vi "GUI.vi"() -> ()   [LabVIEW 2021]
uses:
  UI Data.ctl
  Data.ctl
  <vilib>/Instr/_visa.llb/VISA Configure Serial Port (Instr).vi
  styles/colors.vi
panel:
  in  "Stop button":bool
  in  "Run button":bool
  in  "Settings button":bool
  out "Console":string
  in  "Serial communication\n settings":T1={"COM"="", "baud rate"=115200, "data bits"=8, "parity"=enum."None", "stop bits"=10, "flow control"=enum."None", "delay"=50} {"stop bits" items=["1.0"=10, "1.5"=15, "2.0"=20]; "baud rate" max=921600; "data bits" max=16}
  in  "Paths":bool
  in  "Save button":bool
  in  "Path: 4.9.12.XXXX":path=path "C:/Users/ken_X/Documents/LabVIEW projects/Project-A/outset-medical/4.9.12.6034"
  in  "Path: Android OS":path=path "C:/Users/ken_X/Documents/LabVIEW projects/Project-A/outset-medical/Android OS"
  # "Serial communication\n settings"
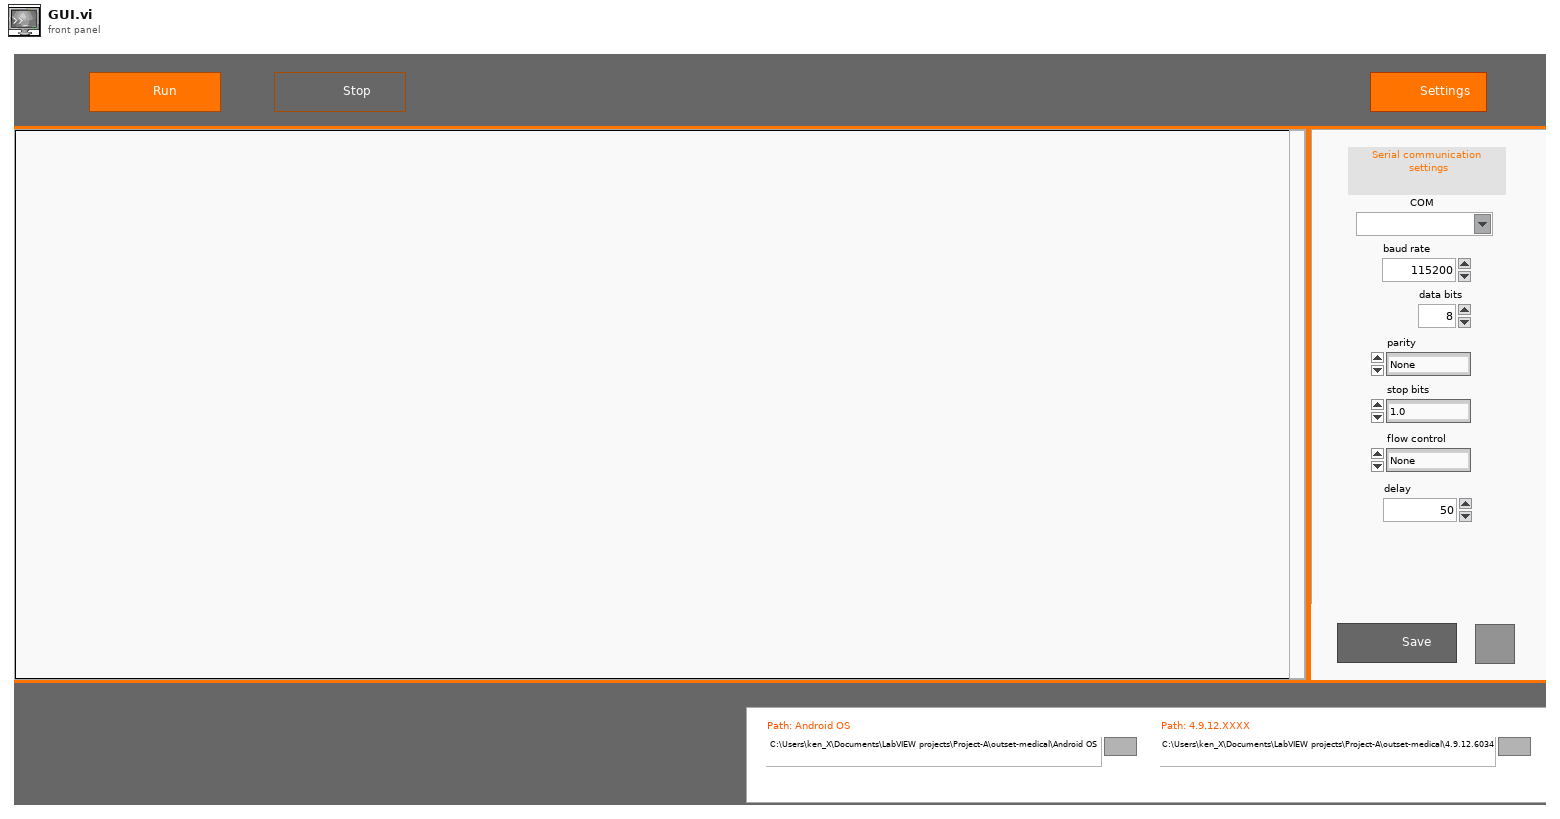
[diagram p1: front panel]
types:
  T1 = cluster{"COM":refnum<visa-resource-name>, "baud rate":u32, "data bits":u8, "parity":enum16{"None", "Odd", "Even", "Mark", "Space"}, "stop bits":u16, "flow control":enum16{"None", "XON/XOFF", "RTS/CTS", "DTR/DSR"}, "delay":u16}
  T2 = typedef "Data.ctl" = cluster{"Console":refnum<vi>, "COM":refnum<visa-resource-name>, "delay":u32, "error in":errorcluster}
  T3 = enum8{"Enabled", "Disabled", "Disabled and Grayed Out"}
  T4 = typedef "UI Data.ctl" = cluster{"settings splitter":refnum<vi>, "footer splitter":refnum<vi>, "Serial communication\n settings":refnum<vi>, "Path: Android OS":refnum<vi>, "Path: 4.9.12.XXXX":refnum<vi>}
  T5 = cluster{"primary color":u32, "secondary color":u32, "accent color":u32, "background color":u32, "accent s color":u32}
  T6 = cluster{"accent s color":u32, "accent s color":u32}
  T7 = cluster{"accent s color":u32, "accent color":u32}
  T8 = cluster{"primary color":u32, "primary color":u32}
  T9 = cluster{"secondary color":u32, "secondary color":u32}
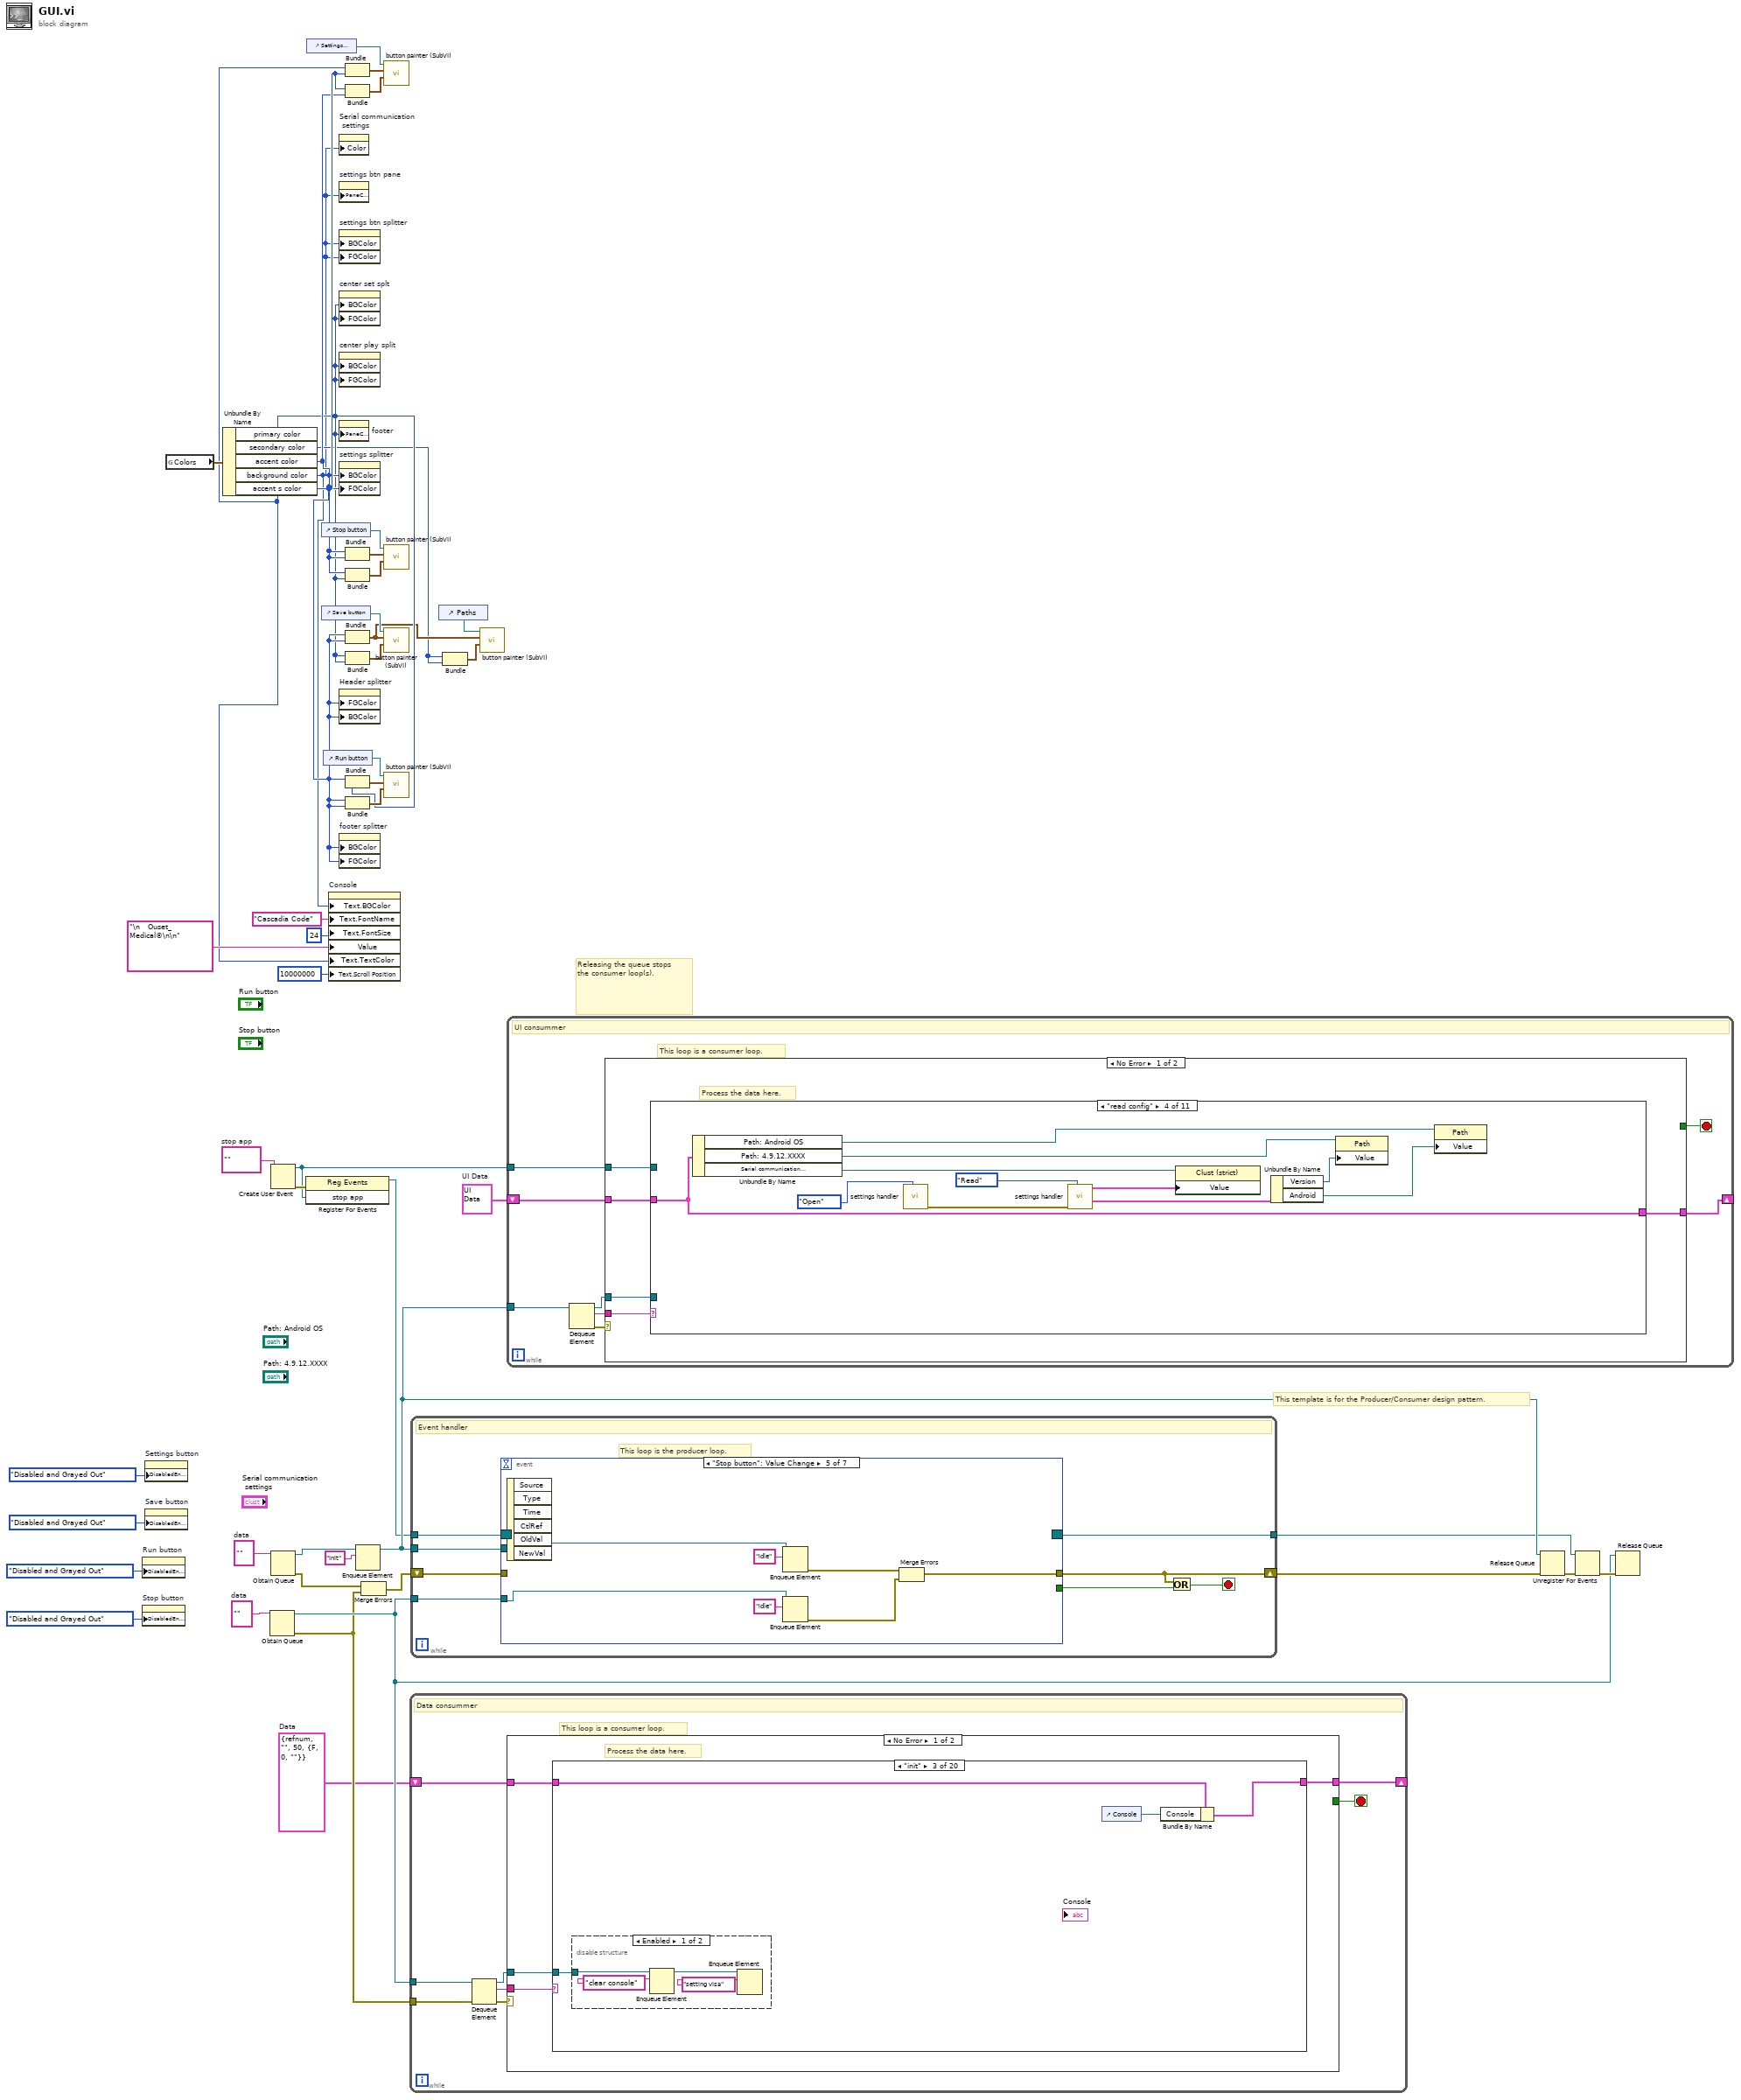
[diagram p0: block diagram]
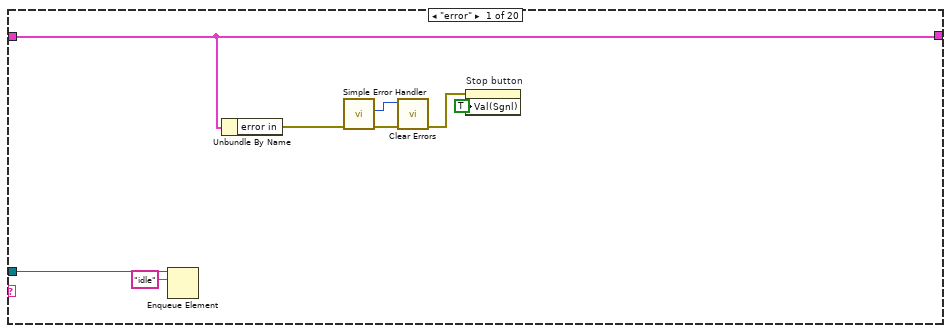
[diagram p2: hidden frame]
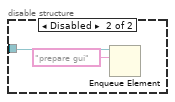
[diagram p4: hidden frame]
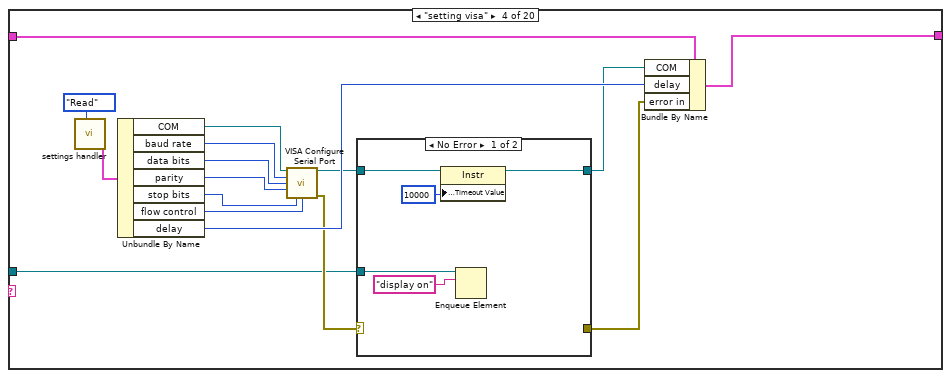
[diagram p5: hidden frame]
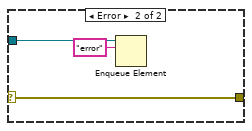
[diagram p6: hidden frame]
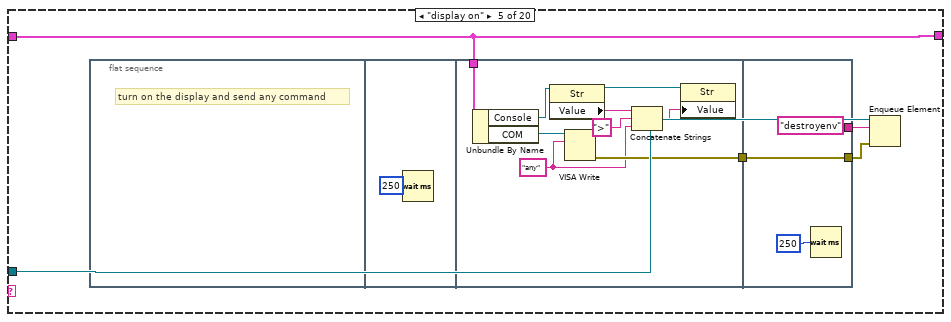
[diagram p7: hidden frame]
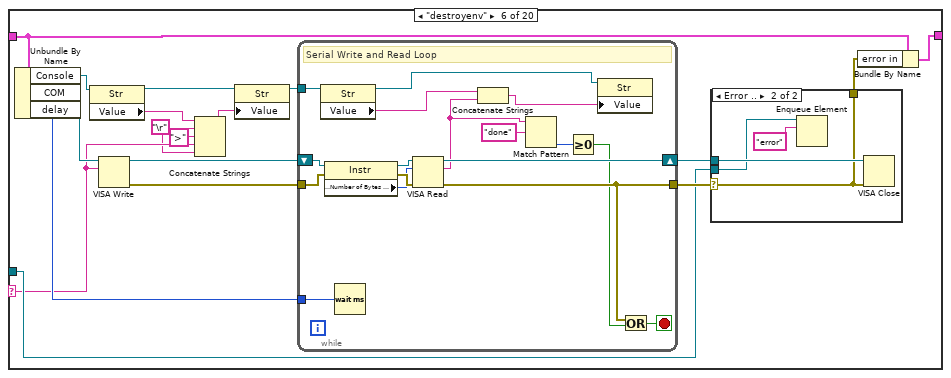
[diagram p8: hidden frame]
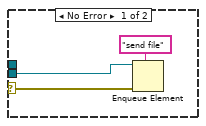
[diagram p9: hidden frame]
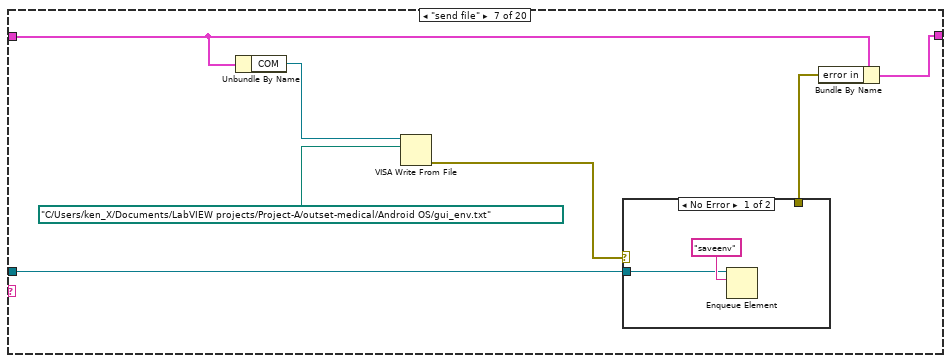
[diagram p10: hidden frame]
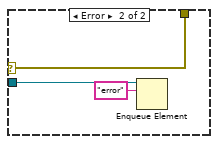
[diagram p11: hidden frame]
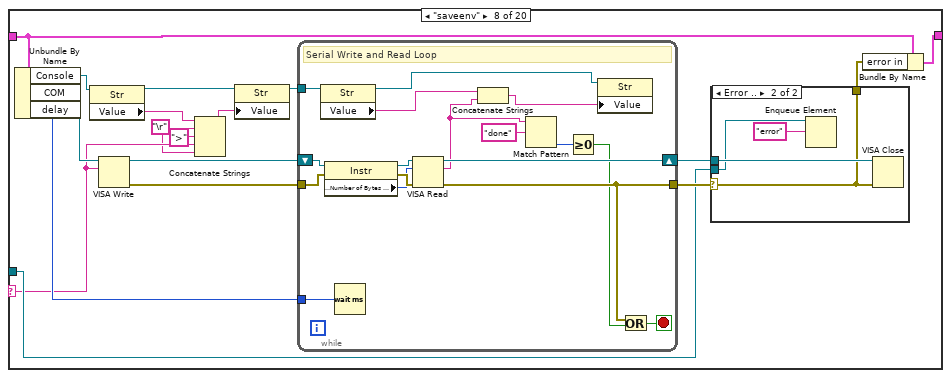
[diagram p12: hidden frame]
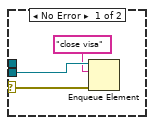
[diagram p13: hidden frame]
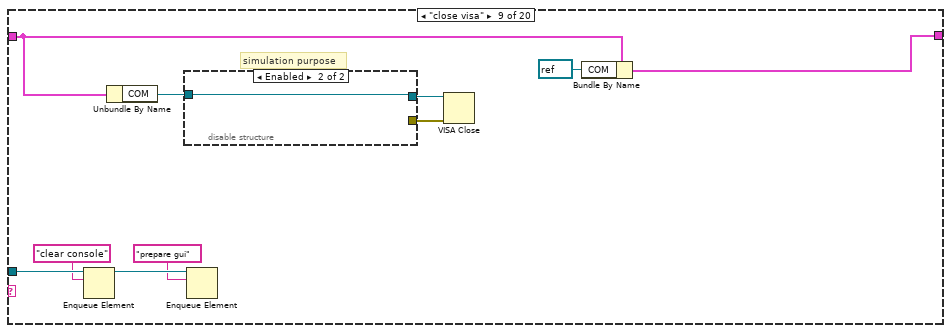
[diagram p14: hidden frame]
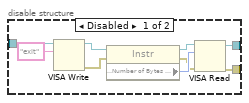
[diagram p15: hidden frame]
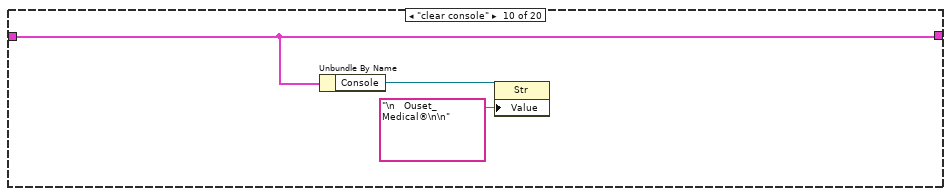
[diagram p16: hidden frame]
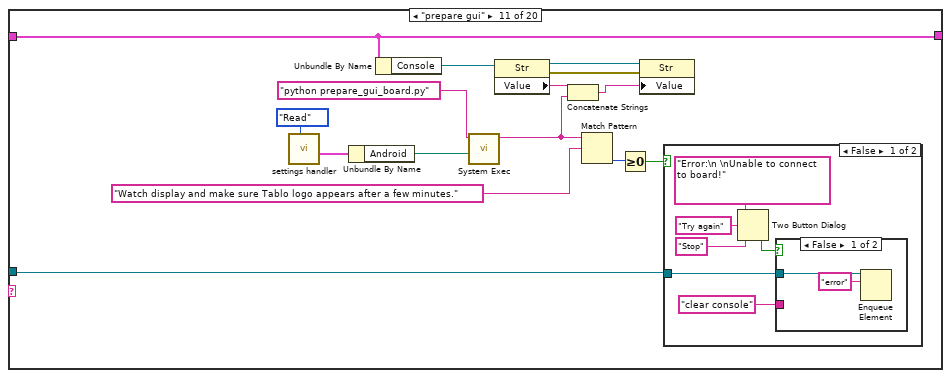
[diagram p17: hidden frame]
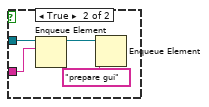
[diagram p18: hidden frame]
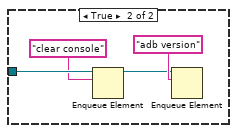
[diagram p19: hidden frame]
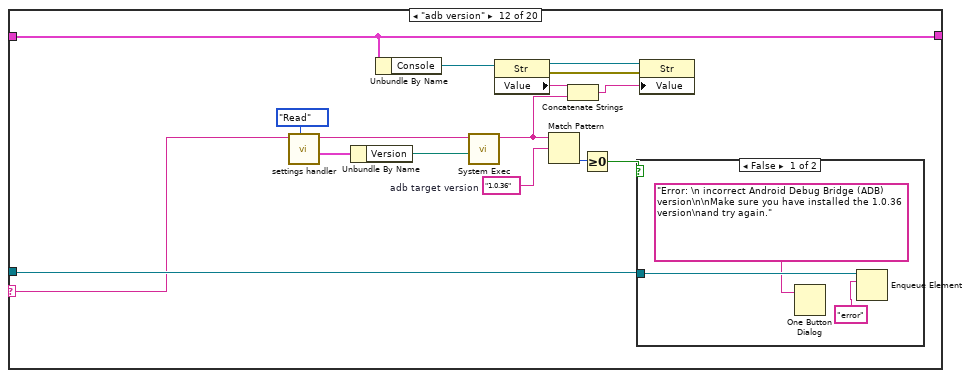
[diagram p20: hidden frame]
diagram:
  w14 = T2 {"Console"=refnum, "COM"="", "delay"=50, "error in"={"status"=FALSE, "code"=0, "source"=""}}  # Data
  w22 = ""  # data
  w38 = ""  # stop app
  w42 = T4 {"settings splitter"=refnum, "footer splitter"=refnum, "Serial communication\n settings"=refnum, "Path: Android OS"=refnum, "Path: 4.9.12.XXXX"=refnum}  # UI Data
  w39 = ""  # data
  # "Releasing the queue stops the consumer loop(s)."
  # "This template is for the Producer/Consumer design pattern."
  n1 = property on="Run button" class="Bool (strict)"("DisabledEnum"=T3."Disabled and Grayed Out" ("Disabled")) -> ()  [unwired: 2 in, 2 out]
  n2 = property on="Stop button" class="Bool (strict)"("DisabledEnum"=T3."Disabled and Grayed Out" ("Disabled")) -> ()  [unwired: 2 in, 2 out]
  n3 = property on="Settings button" class="Bool (strict)"("DisabledEnum"=T3."Disabled and Grayed Out" ("Disabled")) -> ()  [unwired: 2 in, 2 out]
  n4 = property on="Save button" class="Bool (strict)"("DisabledEnum"=T3."Disabled and Grayed Out" ("Disabled")) -> ()  [unwired: 2 in, 2 out]
  n5 = global read "colors.vi" "Colors"() -> (w47:T5)
  n6 = Unbundle By Name(w47) -> ("primary color"=w7:u32, "secondary color"=w3:u32, "accent color"=w8:u32, "background color"=w1:u32, "accent s color"=w10:u32)
  n7 = Obtain Queue(element data type=w22) -> (queue out=w18:refnum<queue>, error out=w17:errorcluster)  [unwired: 4 in, 1 out]
  n8 = Create User Event(user event datatype=w38) -> (user event=w36:refnum<user-event>, error out=w37:errorcluster)  [unwired: 1 in]
  n9 = Obtain Queue(element data type=w39) -> (queue out=w45:refnum<queue>, error out=w21:errorcluster)  [unwired: 4 in, 1 out]
  n10 = register-events(error in=w37, w36) -> (reference out=w35:refnum<event-registration>)  [unwired: 1 in, 1 out]
  n11 = control-ref of="Settings button"() -> (w27:refnum<vi>)
  n12 = control-ref of="Stop button"() -> (w25:refnum<vi>)
  n13 = control-ref of="Save button"() -> (w26:refnum<vi>)
  n14 = control-ref of="Run button"() -> (w32:refnum<vi>)
  n15 = property on="Console" class="Str"("Text.BGColor"=w1, "Text.FontName"="Cascadia Code" ("Text.Font:Name"), "Text.FontSize"=u32 24 ("Text.Font:Size"), "Value"="\n   Ouset_Medical®\n\n" ("Console"), "Text.TextColor"=w10, "Text.Scroll Position"=u32 10000000) -> ()  [unwired: 2 in, 2 out]
  n16 = property on="Serial communication\n settings" class="Clust (strict)"("Color"=w1) -> ()  [unwired: 2 in, 2 out]
  n17 = property on="settings btn pane" class="Pane"("PaneColor"=w1) -> ()  [unwired: 2 in, 2 out]
  n18 = property on="settings btn splitter" class="Splitter"("BGColor"=w1, "FGColor"=w1) -> ()  [unwired: 2 in, 2 out]
  n19 = property on="center set splt" class="Splitter"("BGColor"=w7, "FGColor"=w7) -> ()  [unwired: 2 in, 2 out]
  n20 = property on="center play split" class="Splitter"("BGColor"=w7, "FGColor"=w7) -> ()  [unwired: 2 in, 2 out]
  n21 = property on="footer" class="Pane"("PaneColor"=w7) -> ()  [unwired: 2 in, 2 out]
  n22 = property on="settings splitter" class="Splitter"("BGColor"=w8, "FGColor"=w8) -> ()  [unwired: 2 in, 2 out]
  n23 = property on="Header splitter" class="Splitter"("FGColor"=w8, "BGColor"=w8) -> ()  [unwired: 2 in, 2 out]
  n24 = property on="footer splitter" class="Splitter"("BGColor"=w8, "FGColor"=w8) -> ()  [unwired: 2 in, 2 out]
  n25 = Bundle("accent s color"=w10, "accent s color"=w10) -> (w29:T6)  [unwired: 1 in]
  n26 = Bundle("accent s color"=w10, "accent color"=w8) -> (w28:T7)  [unwired: 1 in]
  n27 = Bundle("accent color"=w8, "accent color"=w8) -> (w23:cluster{"accent color":u32, "accent color":u32})  [unwired: 1 in]
  n28 = Bundle("accent color"=w8, "primary color"=w7) -> (w24:cluster{"accent color":u32, "primary color":u32})  [unwired: 1 in]
  n29 = Bundle("accent color"=w8, "accent color"=w8) -> (w5:cluster{"accent color":u32, "accent color":u32})  [unwired: 1 in]
  n30 = Bundle("primary color"=w7, "primary color"=w7) -> (w4:T8)  [unwired: 1 in]
  n31 = Bundle("accent color"=w8, "primary color"=w7) -> (w30:cluster{"accent color":u32, "primary color":u32})  [unwired: 1 in]
  n32 = Bundle("accent color"=w8, "accent color"=w8) -> (w31:cluster{"accent color":u32, "accent color":u32})  [unwired: 1 in]
  n33 = Enqueue Element(queue=w45, element="init") -> (queue out=w44:refnum<queue>)  [unwired: 2 in, 2 out]
  n34 = Merge Errors(w21, w17) -> (w20:errorcluster)
  n35 = call "button painter (SubVI).vi"("Off state"=w28, "On state"=w29, "Button ref in"=w27) -> ()  [unwired: 9 in]
  n36 = call "button painter (SubVI).vi"("Off state"=w24, "On state"=w23, "Button ref in"=w25) -> ()  [unwired: 9 in]
  n37 = call "button painter (SubVI).vi"("Off state"=w4, "On state"=w5, "Button ref in"=w26) -> ()  [unwired: 9 in]
  n38 = call "button painter (SubVI).vi"("Off state"=w31, "On state"=w30, "Button ref in"=w32) -> ()  [unwired: 9 in]
  n39 = while {
    tunnel: w18 -> [w55]
    tunnel: w17 -> [w50]
    shift-right: [w48] -> _
    shift-left: w14 -> [w49]
    stop <- w53 stop-if-true
    # "This loop is a consumer loop."
    # "Data consummer"
    n40 = Dequeue Element(queue=w55, error in (no error)=w50) -> (queue out=w51:refnum<queue>, element=w52:string, error out=w54:errorcluster)  [unwired: 1 in, 1 out]
    n41 = case shown="No Error" w54 {
      tunnel: [_ TRUE] -> w53
      tunnel: w52 -> [w59 _]
      tunnel: w51 -> [w58 _]
      tunnel: w49 -> [w57 _]
      tunnel: [w56 _] -> w48
      frame No Error {
        # "Process the data here."
        n42 = case shown="\"init\"" w59 {
          selector: w59 -> [_ _ _ _ _ w128 _ w182 _ _ _ w271 _ _ _ _ w376 _ _ _]
          tunnel: w58 -> [w61 _ w72 w82 w106 w133 w167 w187 w220 _ w240 w272 w292 w321 w342 w355 w377 w388 w391 _]
          tunnel: w57 -> [w63 w68 w71 w88 w103 w123 w165 w177 w226 w238 w251 w282 w302 w331 w347 w365 w383 w389 w392 w403]
          tunnel: [w63 w68 w69 w87 w103 w122 w164 w176 w225 w238 w251 w282 w302 w331 w347 w365 w383 w389 w392 w403] -> w56
          frame "error" {
            n43 = Enqueue Element(queue=w61, element="idle") -> ()  [unwired: 2 in, 3 out]
            n44 = Unbundle By Name(w63) -> ("error in"=w62:errorcluster)
            n45 = call <vilib>:"Simple Error Handler.vi"("error in (no error)"=w62) -> ("code out"=w66:i32, "error out"=w67:errorcluster)  [unwired: 4 in, 3 out]
            n46 = call <vilib>:"Clear Errors.vi"("error in (no error)"=w67, "specific error code to clear (0: all)"=w66) -> ("error out"=w65:errorcluster)  [unwired: 4 in, 1 out]
            n47 = property on="Stop button" class="Bool (strict)"(error in=w65, "Val(Sgnl)"=TRUE ("Value (Signaling)")) -> ()  [unwired: 1 in, 2 out]
          }
          frame "idle", Default {
          }
          frame "init" {
            n48 = disable-structure shown="Enabled" {
              disable-tunnel: w72 -> [w74 w78]
              frame Enabled {
                n49 = Enqueue Element(queue=w74, element="clear console") -> (queue out=w75:refnum<queue>)  [unwired: 2 in, 2 out]
                n50 = Enqueue Element(queue=w75, element="setting visa") -> ()  [unwired: 2 in, 3 out]
              }
              frame Disabled {
                n51 = Enqueue Element(queue=w78, element="prepare gui") -> ()  [unwired: 2 in, 3 out]
              }
            }
            n52 = control-ref of="Console"() -> (w70:refnum<vi>)
            n53 = Bundle By Name(cluster=w71, "Console"=w70) -> (w69:T2)
          }
          frame "setting visa" {
            n54 = call "settings handler.vi"("Operation"=enum16{"Open", "Write", "Read", "Close"}."Read") -> ("Read"=w93:T1)  [unwired: 8 in, 2 out]
            n55 = Unbundle By Name(w93) -> ("COM"=w92:refnum<visa-resource-name>, "baud rate"=w91:u32, "data bits"=w90:u8, "parity"=w89:enum16{"None", "Odd", "Even", "Mark", "Space"}, "stop bits"=w85:u16, "flow control"=w86:enum16{"None", "XON/XOFF", "RTS/CTS", "DTR/DSR"}, "delay"=w84:u16)
            n56 = call-poly "VISA Configure Serial Port"("VISA resource name"=w92, "baud rate (9600)"=w91, "data bits (8)"=w90, "parity (0:none)"=w89, "stop bits (10: 1 bit)"=w85, "flow control (0:none)"=w86) -> ("VISA resource name out"=w81:refnum<visa-resource-name>, "error out"=w83:errorcluster)  [unwired: 4 in, 4 out]
            n57 = case shown="No Error" w83 {
              selector: w83 -> [_ w100]
              tunnel: w82 -> [w99 w102]
              tunnel: w81 -> [w97 _]
              tunnel: [w95 _] -> w80
              tunnel: [_ w100] -> w79
              frame No Error {
                n58 = property class="Instr"(reference=w97, "General Settings:Timeout Value"=u32 10000) -> (reference out=w95:refnum<visa-resource-name>)  [unwired: 1 in, 1 out]
                n59 = Enqueue Element(queue=w99, element="display on") -> ()  [unwired: 2 in, 3 out]
              }
              frame Error {
                n60 = Enqueue Element(queue=w102, element="error") -> ()  [unwired: 2 in, 3 out]
              }
            }
            n61 = Bundle By Name(cluster=w88, "COM"=w80, "delay"=w84, "error in"=w79) -> (w87:T2)
          }
          frame "display on" {
            n62 = flat-sequence {
              tunnel: w103 -> [w117]
              tunnel: [w115] -> w105
              tunnel: [w120] -> w107
              tunnel: w105 -> [w120]
              tunnel: ["destroyenv" ("element")] -> w104
              frame #0 {
                # "turn on the display and send any command"
              }
              frame #1 {
                n63 = Wait (ms)(milliseconds to wait=u32 250) -> ()  [unwired: 1 out]
              }
              frame #2 {
                w109 = "any" ("write buffer")
                n64 = Unbundle By Name(w117) -> ("Console"=w114:refnum<vi>, "COM"=w116:refnum<visa-resource-name>)
                n65 = property class="Str"(reference=w114) -> (reference out=w112:refnum<vi>, "Value"=w113:string)  [unwired: 1 in, 1 out]
                n66 = VISA Write(VISA resource name=w116, write buffer=w109) -> (error out=w115:errorcluster)  [unwired: 1 in, 2 out]
                n67 = Concatenate Strings(w113, ">" ("string"), w109) -> (w111:string)
                n68 = property class="Str"(reference=w112, "Value"=w111) -> ()  [unwired: 1 in, 2 out]
              }
              frame #3 {
                n69 = Wait (ms)(milliseconds to wait=u32 250) -> ()  [unwired: 1 out]
              }
            }
            n70 = Enqueue Element(queue=w106, element=w104, error in (no error)=w107) -> ()  [unwired: 1 in, 3 out]
          }
          frame "destroyenv" {
            w124 = "\r"
            n71 = Unbundle By Name(w123) -> ("Console"=w131:refnum<vi>, "COM"=w134:refnum<visa-resource-name>, "delay"=w132:u32)
            n72 = property class="Str"(reference=w131) -> (reference out=w127:refnum<vi>, "Value"=w130:string)  [unwired: 1 in, 1 out]
            n73 = VISA Write(VISA resource name=w134, write buffer=w128) -> (VISA resource name out=w138:refnum<visa-resource-name>, error out=w137:errorcluster)  [unwired: 1 in, 1 out]
            n74 = Concatenate Strings(w130, w124, ">" ("string"), w128, w124) -> (w126:string)
            n75 = property class="Str"(reference=w127, "Value"=w126) -> (reference out=w125:refnum<vi>)  [unwired: 1 in, 1 out]
            n76 = while {
              shift-right: [w162] -> w135
              shift-left: w138 -> [w156]
              tunnel: [w160] -> w136
              tunnel: w137 -> [w155]
              tunnel: w132 -> [w151]
              tunnel: w125 -> [w150]
              stop <- w161 stop-if-true
              # "Serial Write and Read Loop"
              n77 = property class="Str"(reference=w150) -> (reference out=w149:refnum<vi>, "Value"=w147:string)  [unwired: 1 in, 1 out]
              n78 = property class="Instr"(reference=w156, error in=w155) -> (reference out=w154:refnum<visa-resource-name>, error out=w153:errorcluster, "Serial Settings:Number of Bytes at Serial Port"=w152:u32)
              n79 = Wait (ms)(milliseconds to wait=w151) -> ()  [unwired: 1 out]
              n80 = VISA Read(VISA resource name=w154, byte count=w152, error in (no error)=w153) -> (VISA resource name out=w162:refnum<visa-resource-name>, read buffer=w146:string, error out=w160:errorcluster)  [unwired: 1 out]
              n81 = Concatenate Strings(w147, w146) -> (w148:string)
              n82 = Match Pattern(string=w146, regular expression="done") -> (offset past match=w158:i32)  [unwired: 1 in, 3 out]
              n83 = Greater Or Equal To 0?(x=w158) -> (x >= 0?=w157:bool)
              n84 = property class="Str"(reference=w149, "Value"=w148) -> ()  [unwired: 1 in, 2 out]
              n85 = Or(x=w160, y=w157) -> (x .or. y?=w161:bool)
            }
            n86 = case shown="Error .." w136 {
              selector: w136 -> [w141 w142]
              tunnel: w135 -> [_ w145]
              tunnel: w133 -> [w140 w144]
              tunnel: [_ w142] -> w121
              frame No Error {
                n87 = Enqueue Element(queue=w140, element="send file", error in (no error)=w141) -> ()  [unwired: 1 in, 3 out]
              }
              frame Error {
                n88 = Enqueue Element(queue=w144, element="error") -> ()  [unwired: 2 in, 3 out]
                n89 = VISA Close(VISA resource name=w145, error in (no error)=w142) -> ()  [unwired: 1 out]
              }
            }
            n90 = Bundle By Name(cluster=w123, "error in"=w121) -> (w122:T2)
          }
          frame "send file" {
            n91 = Unbundle By Name(w165) -> ("COM"=w168:refnum<visa-resource-name>)
            n92 = VISA Write From File(10:path "C:/Users/ken_X/Documents/LabVIEW projects/Project-A/outset-medical/Android OS/gui_env.txt" ("file path (use dialog)"), 11:w168) -> (0:w166:errorcluster)  [unwired: 2 in, 2 out]
            n93 = case shown="No Error" w166 {
              selector: w166 -> [_ w172]
              tunnel: w167 -> [w170 w174]
              tunnel: [_ w172] -> w163
              frame No Error {
                n94 = Enqueue Element(queue=w170, element="saveenv") -> ()  [unwired: 2 in, 3 out]
              }
              frame Error {
                n95 = Enqueue Element(queue=w174, element="error") -> ()  [unwired: 2 in, 3 out]
              }
            }
            n96 = Bundle By Name(cluster=w165, "error in"=w163) -> (w164:T2)
          }
          frame "saveenv" {
            w178 = "\r"
            n97 = Unbundle By Name(w177) -> ("Console"=w185:refnum<vi>, "COM"=w188:refnum<visa-resource-name>, "delay"=w186:u32)
            n98 = property class="Str"(reference=w185) -> (reference out=w181:refnum<vi>, "Value"=w184:string)  [unwired: 1 in, 1 out]
            n99 = VISA Write(VISA resource name=w188, write buffer=w182) -> (VISA resource name out=w192:refnum<visa-resource-name>, error out=w191:errorcluster)  [unwired: 1 in, 1 out]
            n100 = Concatenate Strings(w184, w178, ">" ("string"), w182, w178) -> (w180:string)
            n101 = property class="Str"(reference=w181, "Value"=w180) -> (reference out=w179:refnum<vi>)  [unwired: 1 in, 1 out]
            n102 = while {
              shift-right: [w216] -> w189
              shift-left: w192 -> [w210]
              tunnel: [w214] -> w190
              tunnel: w191 -> [w209]
              tunnel: w186 -> [w205]
              tunnel: w179 -> [w204]
              stop <- w215 stop-if-true
              # "Serial Write and Read Loop"
              n103 = property class="Str"(reference=w204) -> (reference out=w203:refnum<vi>, "Value"=w201:string)  [unwired: 1 in, 1 out]
              n104 = property class="Instr"(reference=w210, error in=w209) -> (reference out=w208:refnum<visa-resource-name>, error out=w207:errorcluster, "Serial Settings:Number of Bytes at Serial Port"=w206:u32)
              n105 = Wait (ms)(milliseconds to wait=w205) -> ()  [unwired: 1 out]
              n106 = VISA Read(VISA resource name=w208, byte count=w206, error in (no error)=w207) -> (VISA resource name out=w216:refnum<visa-resource-name>, read buffer=w200:string, error out=w214:errorcluster)  [unwired: 1 out]
              n107 = Concatenate Strings(w201, w200) -> (w202:string)
              n108 = Match Pattern(string=w200, regular expression="done") -> (offset past match=w212:i32)  [unwired: 1 in, 3 out]
              n109 = Greater Or Equal To 0?(x=w212) -> (x >= 0?=w211:bool)
              n110 = property class="Str"(reference=w203, "Value"=w202) -> ()  [unwired: 1 in, 2 out]
              n111 = Or(x=w214, y=w211) -> (x .or. y?=w215:bool)
            }
            n112 = case shown="Error .." w190 {
              selector: w190 -> [w195 w196]
              tunnel: w189 -> [_ w198]
              tunnel: w187 -> [w194 w197]
              tunnel: [_ w196] -> w175
              frame No Error {
                n113 = Enqueue Element(queue=w194, element="close visa", error in (no error)=w195) -> ()  [unwired: 1 in, 3 out]
              }
              frame Error {
                n114 = Enqueue Element(queue=w197, element="error") -> ()  [unwired: 2 in, 3 out]
                n115 = VISA Close(VISA resource name=w198, error in (no error)=w196) -> ()  [unwired: 1 out]
              }
            }
            n116 = Bundle By Name(cluster=w177, "error in"=w175) -> (w176:T2)
          }
          frame "close visa" {
            # "simulation purpose"
            n117 = Enqueue Element(queue=w220, element="clear console") -> (queue out=w218:refnum<queue>)  [unwired: 2 in, 2 out]
            n118 = Unbundle By Name(w226) -> ("COM"=w223:refnum<visa-resource-name>)
            n119 = disable-structure shown="Enabled" {
              disable-tunnel: w223 -> [w235 w236]
              disable-tunnel: [w228 w236] -> w222
              disable-tunnel: [w227 _] -> w221
              frame Disabled {
                n120 = VISA Write(VISA resource name=w235, write buffer="exit") -> (VISA resource name out=w233:refnum<visa-resource-name>, error out=w232:errorcluster)  [unwired: 1 in, 1 out]
                n121 = property class="Instr"(reference=w233, error in=w232) -> (reference out=w230:refnum<visa-resource-name>, error out=w229:errorcluster, "Serial Settings:Number of Bytes at Serial Port"=w231:u32)
                n122 = VISA Read(VISA resource name=w230, byte count=w231, error in (no error)=w229) -> (VISA resource name out=w228:refnum<visa-resource-name>, error out=w227:errorcluster)  [unwired: 2 out]
              }
              frame Enabled {
              }
            }
            n123 = Enqueue Element(queue=w218, element="prepare gui") -> ()  [unwired: 2 in, 3 out]
            n124 = VISA Close(VISA resource name=w222, error in (no error)=w221) -> ()  [unwired: 1 out]
            n125 = Bundle By Name(cluster=w226, "COM"=refnum<visa-resource-name> refnum) -> (w225:T2)
          }
          frame "clear console" {
            n126 = Unbundle By Name(w238) -> ("Console"=w237:refnum<vi>)
            n127 = property class="Str"(reference=w237, "Value"="\n   Ouset_Medical®\n\n") -> ()  [unwired: 1 in, 2 out]
          }
          frame "prepare gui" {
            n128 = call "settings handler.vi"("Operation"=enum16{"Open", "Write", "Read", "Close"}."Read") -> ("Paths read"=w253:cluster{"Android":path, "Version":path})  [unwired: 8 in, 2 out]
            n129 = Unbundle By Name(w253) -> ("Android"=w252:path)
            n130 = Unbundle By Name(w251) -> ("Console"=w250:refnum<vi>)
            n131 = call <vilib>:"System Exec.vi"("working directory"=w252, "command line"="python prepare_gui_board.py") -> ("standard output"=w244:string)  [unwired: 6 in, 3 out]
            n132 = property class="Str"(reference=w250) -> (reference out=w249:refnum<vi>, error out=w246:errorcluster, "Value"=w248:string)  [unwired: 1 in]
            n133 = Concatenate Strings(w248, w244) -> (w247:string)
            n134 = Match Pattern(string=w244, regular expression="Watch display and make sure Tablo logo appears after a few minutes.") -> (offset past match=w242:i32)  [unwired: 1 in, 3 out]
            n135 = Greater Or Equal To 0?(x=w242) -> (x >= 0?=w241:bool)
            n136 = property class="Str"(reference=w249, error in=w246, "Value"=w247) -> ()  [unwired: 2 out]
            n137 = case shown="False" w241 {
              tunnel: w240 -> [w256 w270]
              frame False {
                n138 = Two Button Dialog(message="Error:\n \nUnable to connect to board!", 1:"Stop" ("F button name (\"Cancel\")"), 2:"Try again" ("T button name (\"OK\")")) -> (T button?=w257:bool)
                n139 = case shown="False" w257 {
                  tunnel: w256 -> [w262 w265]
                  tunnel: "clear console" -> [_ w263]
                  frame False {
                    n140 = Enqueue Element(queue=w262, element="error") -> ()  [unwired: 2 in, 3 out]
                  }
                  frame True {
                    n141 = Enqueue Element(queue=w265, element=w263) -> (queue out=w264:refnum<queue>)  [unwired: 2 in, 2 out]
                    n142 = Enqueue Element(queue=w264, element="prepare gui") -> ()  [unwired: 2 in, 3 out]
                  }
                }
              }
              frame True {
                n143 = Enqueue Element(queue=w270, element="clear console") -> (queue out=w268:refnum<queue>)  [unwired: 2 in, 2 out]
                n144 = Enqueue Element(queue=w268, element="adb version") -> ()  [unwired: 2 in, 3 out]
              }
            }
          }
          frame "adb version" {
            w275 = "1.0.36"  # adb target version
            n145 = call "settings handler.vi"("Operation"=enum16{"Open", "Write", "Read", "Close"}."Read") -> ("Paths read"=w284:cluster{"Android":path, "Version":path})  [unwired: 8 in, 2 out]
            n146 = Unbundle By Name(w284) -> ("Version"=w283:path)
            n147 = Unbundle By Name(w282) -> ("Console"=w281:refnum<vi>)
            n148 = call <vilib>:"System Exec.vi"("working directory"=w283, "command line"=w271) -> ("standard output"=w276:string)  [unwired: 6 in, 3 out]
            n149 = property class="Str"(reference=w281) -> (reference out=w280:refnum<vi>, error out=w277:errorcluster, "Value"=w279:string)  [unwired: 1 in]
            n150 = Match Pattern(string=w276, regular expression=w275) -> (offset past match=w274:i32)  [unwired: 1 in, 3 out]
            n151 = Concatenate Strings(w279, w276) -> (w278:string)
            n152 = Greater Or Equal To 0?(x=w274) -> (x >= 0?=w273:bool)
            n153 = case shown="False" w273 {
              tunnel: w272 -> [w288 w290]
              frame False {
                n154 = One Button Dialog(message="Error: \n incorrect Android Debug Bridge (ADB) version\n\nMake sure you have installed the 1.0.36 version\nand try again.") -> ()  [unwired: 1 in, 1 out]
                n155 = Enqueue Element(queue=w288, element="error") -> ()  [unwired: 2 in, 3 out]
              }
              frame True {
                n156 = Enqueue Element(queue=w290, element="adb connect") -> ()  [unwired: 2 in, 3 out]
              }
            }
            n157 = property class="Str"(reference=w280, error in=w277, "Value"=w278) -> ()  [unwired: 2 out]
          }
          frame "adb connect" {
            n158 = call "settings handler.vi"("Operation"=enum16{"Open", "Write", "Read", "Close"}."Read") -> ("Paths read"=w304:cluster{"Android":path, "Version":path})  [unwired: 8 in, 2 out]
            n159 = Unbundle By Name(w304) -> ("Version"=w303:path)
            n160 = Unbundle By Name(w302) -> ("Console"=w301:refnum<vi>)
            n161 = call <vilib>:"System Exec.vi"("working directory"=w303, "command line"="adb connect 10.134.246.252") -> ("standard output"=w296:string)  [unwired: 6 in, 3 out]
            n162 = property class="Str"(reference=w301) -> (reference out=w300:refnum<vi>, error out=w297:errorcluster, "Value"=w299:string)  [unwired: 1 in]
            n163 = Concatenate Strings(w299, w296) -> (w298:string)
            n164 = Match Pattern(string=w296, regular expression="connected") -> (offset past match=w294:i32)  [unwired: 1 in, 3 out]
            n165 = Greater Or Equal To 0?(x=w294) -> (x >= 0?=w293:bool)
            n166 = property class="Str"(reference=w300, error in=w297, "Value"=w298) -> ()  [unwired: 2 out]
            n167 = case shown="False" w293 {
              tunnel: w292 -> [w306 w319]
              frame False {
                n168 = Two Button Dialog(message="Error:\n\nUnable to connect to 10.134.246.252!", 1:"Stop" ("F button name (\"Cancel\")"), 2:"Try again" ("T button name (\"OK\")")) -> (T button?=w311:bool)
                n169 = case shown="False" w311 {
                  tunnel: "clear console" -> [_ w315]
                  tunnel: w306 -> [w312 w314]
                  frame False {
                    n170 = Enqueue Element(queue=w312, element="error") -> ()  [unwired: 2 in, 3 out]
                  }
                  frame True {
                    n171 = Enqueue Element(queue=w314, element=w315) -> (queue out=w316:refnum<queue>)  [unwired: 2 in, 2 out]
                    n172 = Enqueue Element(queue=w316, element="adb connect") -> ()  [unwired: 2 in, 3 out]
                  }
                }
              }
              frame True {
                n173 = Enqueue Element(queue=w319, element="os build") -> ()  [unwired: 2 in, 3 out]
              }
            }
          }
          frame "os build" {
            n174 = call "settings handler.vi"("Operation"=enum16{"Open", "Write", "Read", "Close"}."Read") -> ("Paths read"=w333:cluster{"Android":path, "Version":path})  [unwired: 8 in, 2 out]
            n175 = Unbundle By Name(w333) -> ("Version"=w332:path)
            n176 = Unbundle By Name(w331) -> ("Console"=w330:refnum<vi>)
            n177 = call <vilib>:"System Exec.vi"("working directory"=w332, "command line"="adb shell cat /system/build.prop") -> ("standard output"=w325:string)  [unwired: 6 in, 3 out]
            n178 = property class="Str"(reference=w330) -> (reference out=w329:refnum<vi>, error out=w326:errorcluster, "Value"=w328:string)  [unwired: 1 in]
            n179 = Concatenate Strings(w328, w325) -> (w327:string)
            n180 = Match Pattern(string=w325, regular expression="ouset.osbuild=4.0.0.3") -> (offset past match=w323:i32)  [unwired: 1 in, 3 out]
            n181 = Greater Or Equal To 0?(x=w323) -> (x >= 0?=w322:bool)
            n182 = property class="Str"(reference=w329, error in=w326, "Value"=w327) -> ()  [unwired: 2 out]
            n183 = case shown="False" w322 {
              tunnel: w321 -> [w335 w339]
              frame False {
                n184 = One Button Dialog(message="Error: \nincorrect GUI Operative System version \n\nMake sure the OS build is the 4.0.0.3") -> ()  [unwired: 1 in, 1 out]
                n185 = Enqueue Element(queue=w335, element="error") -> ()  [unwired: 2 in, 3 out]
              }
              frame True {
                n186 = Enqueue Element(queue=w339, element="clear console") -> (queue out=w340:refnum<queue>)  [unwired: 2 in, 2 out]
                n187 = Enqueue Element(queue=w340, element="check screen") -> ()  [unwired: 2 in, 3 out]
              }
            }
          }
          frame "check screen" {
            n188 = Two Button Dialog(message="Realice la siguiente verificación funcional de la pantalla táctil, toque cada esquina \ny verifique que aparecen los siguientes números en cada una de ellas:\n-superior izquierda: 0 (+40 / -0), 0 (+40 / -0)\n-inferior izquierda: 0 (+40 / -0), 768 (+0 / -40)\n-inferior derecha: 1024 (+0 / -40), 768 (+0 / -40)\n-superior derecha: 1024 (+0 / -40), 0 (+40 / -0)\nEl numero aparece en la parte inferior central de la pantalla en cada caso. \nSi el número no coincide favor de comunicarse con el supervisor o el ingeniero.", 1:"¡Abortar!" ("F button name (\"Cancel\")"), 2:"Todo bien" ("T button name (\"OK\")")) -> (T button?=w343:bool)
            n189 = case shown="False" w343 {
              tunnel: w342 -> [w349 w352]
              frame False {
                n190 = Enqueue Element(queue=w349, element="error") -> ()  [unwired: 2 in, 3 out]
              }
              frame True {
                n191 = Enqueue Element(queue=w352, element="clear console") -> (queue out=w351:refnum<queue>)  [unwired: 2 in, 2 out]
                n192 = Enqueue Element(queue=w351, element="prepare gui") -> ()  [unwired: 2 in, 3 out]
              }
            }
          }
          frame "load gui" {
            n193 = call "settings handler.vi"("Operation"=enum16{"Open", "Write", "Read", "Close"}."Read") -> ("Paths read"=w367:cluster{"Android":path, "Version":path})  [unwired: 8 in, 2 out]
            n194 = Unbundle By Name(w367) -> ("Version"=w366:path)
            n195 = Unbundle By Name(w365) -> ("Console"=w364:refnum<vi>)
            n196 = call <vilib>:"System Exec.vi"("working directory"=w366, "command line"="cmd /C Load_GUI.bat") -> ("standard output"=w359:string)  [unwired: 6 in, 3 out]
            n197 = property class="Str"(reference=w364) -> (reference out=w363:refnum<vi>, error out=w360:errorcluster, "Value"=w362:string)  [unwired: 1 in]
            n198 = Concatenate Strings(w362, w359) -> (w361:string)
            n199 = Match Pattern(string=w359, regular expression="Success") -> (offset past match=w357:i32)  [unwired: 1 in, 3 out]
            n200 = Greater Or Equal To 0?(x=w357) -> (x >= 0?=w356:bool)
            n201 = property class="Str"(reference=w363, error in=w360, "Value"=w361) -> ()  [unwired: 2 out]
            n202 = case shown="False" w356 {
              tunnel: w355 -> [w370 w374]
              frame False {
                n203 = One Button Dialog(message="Error:  loading the GUI", button name ("OK")="Abort") -> ()  [unwired: 1 out]
                n204 = Enqueue Element(queue=w370, element="error") -> ()  [unwired: 2 in, 3 out]
              }
              frame True {
                n205 = Enqueue Element(queue=w374, element="adb reboot") -> ()  [unwired: 2 in, 3 out]
              }
            }
          }
          frame "adb reboot" {
            n206 = call "settings handler.vi"("Operation"=enum16{"Open", "Write", "Read", "Close"}."Read") -> ("Paths read"=w385:cluster{"Android":path, "Version":path})  [unwired: 8 in, 2 out]
            n207 = Unbundle By Name(w385) -> ("Version"=w384:path)
            n208 = Unbundle By Name(w383) -> ("Console"=w382:refnum<vi>)
            n209 = call <vilib>:"System Exec.vi"("working directory"=w384, "command line"=w376) -> ()  [unwired: 6 in, 4 out]
            n210 = property class="Str"(reference=w382) -> (reference out=w381:refnum<vi>, error out=w378:errorcluster, "Value"=w380:string)  [unwired: 1 in]
            n211 = Concatenate Strings(w380) -> (w379:string)
            n212 = property class="Str"(reference=w381, error in=w378, "Value"=w379) -> ()  [unwired: 2 out]
            n213 = Enqueue Element(queue=w377, element="display reboot") -> ()  [unwired: 2 in, 3 out]
          }
          frame "display reboot" {
            # "turn off display"
            # "turn on the display"
            n214 = Enqueue Element(queue=w388, element="update media") -> ()  [unwired: 2 in, 3 out]
          }
          frame "update media" {
            n215 = Enqueue Element(queue=w391, element="end") -> ()  [unwired: 2 in, 3 out]
            n216 = call "settings handler.vi"("Operation"=enum16{"Open", "Write", "Read", "Close"}."Read") -> ("Paths read"=w401:cluster{"Android":path, "Version":path})  [unwired: 8 in, 2 out]
            n217 = Unbundle By Name(w401) -> ("Version"=w400:path)
            n218 = Unbundle By Name(w392) -> ("Console"=w399:refnum<vi>)
            n219 = call <vilib>:"System Exec.vi"("working directory"=w400, "command line"="python Update_Media.py") -> ("standard output"=w393:string)  [unwired: 6 in, 3 out]
            n220 = property class="Str"(reference=w399) -> (reference out=w398:refnum<vi>, error out=w395:errorcluster, "Value"=w397:string)  [unwired: 1 in]
            n221 = Concatenate Strings(w397, w393) -> (w396:string)
            n222 = property class="Str"(reference=w398, error in=w395, "Value"=w396) -> ()  [unwired: 2 out]
          }
          frame "end" {
            n223 = flat-sequence {
              frame #0 {
                n224 = One Button Dialog(message="¡Instalación terminada!") -> ()  [unwired: 1 in, 1 out]
              }
              frame #1 {
                n225 = property on="Stop button" class="Bool (strict)"("Val(Sgnl)"=TRUE ("Value (Signaling)")) -> ()  [unwired: 2 in, 2 out]
              }
            }
          }
        }
      }
      frame Error {
        # "Return true in any case that should stop the loop."
      }
    }
  }
  n226 = while {
    shift-right: [w411] -> w46
    shift-left: w20 -> [w413]
    tunnel: w44 -> [w414]
    tunnel: w35 -> [w410]
    tunnel: [w408] -> w33
    tunnel: w18 -> [w407]
    stop <- w412 stop-if-true
    # "This loop is the producer loop."
    # "Event handler"
    n227 = event shown="[4] \"Stop button\": Value Change" {
      selector: w410 -> [_ _ _ _ _ _ _]
      dyn-events: [_ _ _ _ _ _ _] -> w408
      timeout: _ -> [_ _ _ _ _ _ _]
      tunnel: w414 -> [w418 w431 w442 w453 w459 w468 _]
      tunnel: w413 -> [w417 w430 w443 w455 _ w465 w469]
      tunnel: [w416 w429 w440 w452 w460 w464 w469] -> w411
      tunnel: [_ _ _ _ _ _ TRUE] -> w409
      tunnel: w407 -> [_ _ _ w456 w458 _ _]
      event "Settings button": Value Change {
        n228 = event-data() -> ("NewVal"=w415:bool)  [unwired: 1 in]
        n229 = case shown="False" w415 {
          tunnel: w418 -> [w421 w427]
          tunnel: w417 -> [w423 w426]
          tunnel: [w420 w425] -> w416
          frame False {
            n230 = Enqueue Element(queue=w421, element="close settings", error in (no error)=w423) -> (error out=w420:errorcluster)  [unwired: 1 in, 2 out]
            n231 = property on="Paths" class="Bool (strict)"("Val(Sgnl)"=FALSE ("Value (Signaling)")) -> ()  [unwired: 2 in, 2 out]
          }
          frame True {
            n232 = Enqueue Element(queue=w427, element="open settings", error in (no error)=w426) -> (error out=w425:errorcluster)  [unwired: 1 in, 2 out]
          }
        }
      }
      event "Paths": Value Change {
        n233 = event-data() -> ("NewVal"=w428:bool)  [unwired: 1 in]
        n234 = case shown="True" w428 {
          tunnel: w431 -> [w432 w439]
          tunnel: w430 -> [w434 w438]
          tunnel: [w435 w437] -> w429
          frame False {
            n235 = Enqueue Element(queue=w432, element="close paths", error in (no error)=w434) -> (error out=w435:errorcluster)  [unwired: 1 in, 2 out]
          }
          frame True {
            n236 = Enqueue Element(queue=w439, element="open paths", error in (no error)=w438) -> (error out=w437:errorcluster)  [unwired: 1 in, 2 out]
          }
        }
      }
      event "Save button": Value Change {
        n237 = event-data() -> ("NewVal"=w441:bool)  [unwired: 1 in, 2 out]
        n238 = case shown="True" w441 {
          tunnel: w442 -> [_ w448]
          tunnel: w443 -> [w444 w447]
          tunnel: [w444 w446] -> w440
          frame False {
          }
          frame True {
            n239 = Enqueue Element(queue=w448, element="save config", error in (no error)=w447) -> (error out=w446:errorcluster)  [unwired: 1 in, 2 out]
          }
        }
      }
      event "Run button": Value Change {
        n240 = event-data() -> ()  [unwired: 1 in, 6 out]
        n241 = Enqueue Element(queue=w453, element="running") -> (error out=w450:errorcluster)  [unwired: 2 in, 2 out]
        n242 = Enqueue Element(queue=w456, element="init", error in (no error)=w455) -> (error out=w451:errorcluster)  [unwired: 1 in, 2 out]
        n243 = Merge Errors(w450, w451) -> (w452:errorcluster)
      }
      event "Stop button": Value Change {
        n244 = event-data() -> ()  [unwired: 1 in, 6 out]
        n245 = Enqueue Element(queue=w459, element="idle") -> (error out=w462:errorcluster)  [unwired: 2 in, 2 out]
        n246 = Enqueue Element(queue=w458, element="idle") -> (error out=w463:errorcluster)  [unwired: 2 in, 2 out]
        n247 = Merge Errors(w462, w463) -> (w460:errorcluster)
      }
      event Panel Close? {
        n248 = event-data() -> ()  [unwired: 1 in, 3 out]
        n249 = Enqueue Element At Opposite End(queue=w468, element="confirm quit", error in (no error)=w465) -> (error out=w464:errorcluster)  [unwired: 1 in, 2 out]
        n250 = event-data("Discard?"=TRUE) -> ()  [unwired: 1 in, 1 out]
      }
      event User Event {
        n251 = event-data() -> ()  [unwired: 1 in, 3 out]
      }
    }
    n252 = Or(x=w411, y=w409) -> (x .or. y?=w412:bool)
  }
  n253 = control-ref of="Paths"() -> (w6:refnum<vi>)
  n254 = Bundle("secondary color"=w3, "secondary color"=w3) -> (w2:T9)  [unwired: 1 in]
  n255 = call "button painter (SubVI).vi"("Off state"=w2, "On state"=w5, "Button ref in"=w6) -> ()  [unwired: 9 in]
  n256 = while {
    tunnel: w44 -> [w478]
    shift-right: [w473] -> _
    shift-left: w42 -> [w474]
    tunnel: w36 -> [w471]
    stop <- w476 stop-if-true
    # "This loop is a consumer loop."
    # "UI consummer"
    n257 = Dequeue Element(queue=w478) -> (queue out=w472:refnum<queue>, element=w475:string, error out=w477:errorcluster)  [unwired: 2 in, 1 out]
    n258 = case shown="No Error" w477 {
      tunnel: [_ TRUE] -> w476
      tunnel: w475 -> [w483 _]
      tunnel: w474 -> [w482 _]
      tunnel: [w481 _] -> w473
      tunnel: w472 -> [w480 _]
      tunnel: w471 -> [w479 _]
      frame No Error {
        # "Process the data here."
        n259 = case shown="\"read config\"" w483 {
          tunnel: w482 -> [w494 w506 w510 w518 w532 w534 w540 w551 w558 w565 w572]
          tunnel: [w493 w506 w510 w518 w532 w534 w540 w551 w558 w565 w572] -> w481
          tunnel: w480 -> [w491 _ _ _ _ _ _ _ _ w562 _]
          tunnel: w479 -> [_ _ _ _ _ _ _ _ _ _ w571]
          frame "init", Default {
            n260 = Enqueue Element(queue=w491, element="read config") -> (queue out=w486:refnum<queue>, error out=w488:errorcluster)  [unwired: 2 in, 1 out]
            n261 = Enqueue Element(queue=w486, element="idle", error in (no error)=w488) -> ()  [unwired: 1 in, 3 out]
            n262 = control-ref of="footer splitter"() -> (w492:refnum<vi>)
            n263 = control-ref of="Serial communication\n settings"() -> (w489:refnum<vi>)
            n264 = control-ref of="Path: Android OS"() -> (w485:refnum<vi>)
            n265 = control-ref of="Path: 4.9.12.XXXX"() -> (w484:refnum<vi>)
            n266 = control-ref of="settings splitter"() -> (w495:refnum<vi>)
            n267 = Bundle By Name(cluster=w494, "settings splitter"=w495, "footer splitter"=w492, "Serial communication\n settings"=w489, "Path: Android OS"=w485, "Path: 4.9.12.XXXX"=w484) -> (w493:T4)
          }
          frame "idle" {
            n268 = property on="Save button" class="Bool (strict)"("DisabledEnum"=T3."Enabled" ("Disabled"), "Value"=FALSE ("Save button")) -> ()  [unwired: 2 in, 2 out]
            n269 = property on="Settings button" class="Bool (strict)"("DisabledEnum"=T3."Enabled" ("Disabled"), "Val(Sgnl)"=FALSE ("Settings")) -> ()  [unwired: 2 in, 2 out]
            n270 = property on="Run button" class="Bool (strict)"("DisabledEnum"=T3."Enabled" ("Disabled"), "Value"=FALSE ("Save button")) -> ()  [unwired: 2 in, 2 out]
            n271 = property on="Stop button" class="Bool (strict)"("DisabledEnum"=T3."Disabled" ("Disabled"), "Value"=FALSE ("Save button")) -> ()  [unwired: 2 in, 2 out]
            n272 = property on="Paths" class="Bool (strict)"("DisabledEnum"=T3."Enabled" ("Disabled"), "Val(Sgnl)"=FALSE ("Paths")) -> ()  [unwired: 2 in, 2 out]
          }
          frame "running" {
            n273 = property on="Run button" class="Bool (strict)"("DisabledEnum"=T3."Disabled" ("Disabled")) -> ()  [unwired: 2 in, 2 out]
            n274 = property on="Stop button" class="Bool (strict)"("Value"=TRUE ("Stop button"), "DisabledEnum"=T3."Enabled" ("Disabled")) -> ()  [unwired: 2 in, 2 out]
          }
          frame "read config" {
            n275 = Unbundle By Name(w518) -> ("Path: Android OS"=w512:refnum<vi>, "Path: 4.9.12.XXXX"=w515:refnum<vi>, "Serial communication\n settings"=w517:refnum<vi>)
            n276 = call "settings handler.vi"("Operation"=enum16{"Open", "Write", "Read", "Close"}."Open") -> ("Error Out"=w521:errorcluster)  [unwired: 8 in, 2 out]
            n277 = call "settings handler.vi"("Operation"=enum16{"Open", "Write", "Read", "Close"}."Read", "error in (no error)"=w521) -> ("Paths read"=w514:cluster{"Android":path, "Version":path}, "Read"=w516:T1)  [unwired: 7 in, 1 out]
            n278 = property class="Clust (strict)"(reference=w517, "Value"=w516) -> ()  [unwired: 1 in, 2 out]
            n279 = Unbundle By Name(w514) -> ("Version"=w513:path, "Android"=w511:path)
            n280 = property class="Path"(reference=w515, "Value"=w513) -> ()  [unwired: 1 in, 2 out]
            n281 = property class="Path"(reference=w512, "Value"=w511) -> ()  [unwired: 1 in, 2 out]
          }
          frame "save config" {
            n282 = Unbundle By Name(w532) -> ("Serial communication\n settings"=w531:refnum<vi>, "Path: Android OS"=w526:refnum<vi>, "Path: 4.9.12.XXXX"=w525:refnum<vi>)
            n283 = property on="Save button" class="Bool (strict)"("Value"=FALSE ("Save button")) -> ()  [unwired: 2 in, 2 out]
            n284 = property class="Clust (strict)"(reference=w531) -> ("Value"=w530:T1)  [unwired: 1 in, 2 out]
            n285 = property class="Path"(reference=w526) -> ("Value"=w524:path)  [unwired: 1 in, 2 out]
            n286 = property class="Path"(reference=w525) -> ("Value"=w523:path)  [unwired: 1 in, 2 out]
            n287 = Bundle("Value"=w524, "Value"=w523) -> (w522:cluster{"Value":path, "Value":path})  [unwired: 1 in]
            n288 = call "settings handler.vi"("Operation"=enum16{"Open", "Write", "Read", "Close"}."Write", "Paths write"=w522, "Write"=w530) -> ("Error Out"=w527:errorcluster)  [unwired: 6 in, 2 out]
            n289 = case shown="No Error" w527 {
              frame No Error {
                n290 = One Button Dialog(message="¡Se ha guardado con éxito!") -> ()  [unwired: 1 in, 1 out]
              }
              frame Error {
              }
            }
          }
          frame "open settings" {
            n291 = Unbundle By Name(w534) -> ("settings splitter"=w536:refnum<vi>, "footer splitter"=w535:refnum<vi>)
            n292 = property class="Splitter"(reference=w535) -> ("Width"=w539:u32)  [unwired: 1 in, 2 out]
            n293 = Subtract(x=w539, y=u32 240) -> (x-y=w538:u32)
            n294 = property class="Splitter"(reference=w536, "Position"=w538) -> ()  [unwired: 1 in, 2 out]
          }
          frame "close settings" {
            n295 = Unbundle By Name(w540) -> ("settings splitter"=w542:refnum<vi>, "footer splitter"=w541:refnum<vi>)
            n296 = property class="Splitter"(reference=w541) -> ("Width"=w545:u32)  [unwired: 1 in, 2 out]
            n297 = Subtract(x=w545, y=u32 6) -> (x-y=w544:u32)
            n298 = property class="Splitter"(reference=w542, "Position"=w544) -> ()  [unwired: 1 in, 2 out]
          }
          frame "open paths" {
            n299 = control-ref of="This VI"() -> (w550:refnum<vi>)
            n300 = Unbundle By Name(w551) -> ("footer splitter"=w552:refnum<vi>)
            n301 = property class="VI"(reference=w550) -> ("Panel"=w549:refnum<vi>)  [unwired: 1 in, 2 out]
            n302 = property class="Pnl"(reference=w549) -> ("Height"=w548:u32)  [unwired: 1 in, 2 out]
            n303 = Subtract(x=w548, y=u32 125) -> (x-y=w546:u32)
            n304 = property class="Splitter"(reference=w552, "Position"=w546) -> ()  [unwired: 1 in, 2 out]
          }
          frame "close paths" {
            n305 = control-ref of="This VI"() -> (w557:refnum<vi>)
            n306 = Unbundle By Name(w558) -> ("footer splitter"=w559:refnum<vi>)
            n307 = property class="VI"(reference=w557) -> ("Panel"=w556:refnum<vi>)  [unwired: 1 in, 2 out]
            n308 = property class="Pnl"(reference=w556) -> ("Height"=w555:u32)  [unwired: 1 in, 2 out]
            n309 = Subtract(x=w555, y=u32 28) -> (x-y=w554:u32)
            n310 = property class="Splitter"(reference=w559, "Position"=w554) -> ()  [unwired: 1 in, 2 out]
          }
          frame "confirm quit" {
            n311 = Two Button Dialog(message="¿Seguro que quiere cerrar\nla aplicación?", 1:"Cancelar" ("F button name (\"Cancel\")"), 2:"Si" ("T button name (\"OK\")")) -> (T button?=w564:bool)
            n312 = case shown="True" w564 {
              tunnel: w562 -> [_ w567]
              frame False {
              }
              frame True {
                n313 = Enqueue Element At Opposite End(queue=w567, element="exit" ("Message")) -> ()  [unwired: 2 in, 3 out]
              }
            }
          }
          frame "exit" {
            n314 = call "settings handler.vi"("Operation"=enum16{"Open", "Write", "Read", "Close"}."Close") -> ("Error Out"=w569:errorcluster)  [unwired: 8 in, 2 out]
            n315 = Generate User Event(user event=w571, event data cluster="stop app" ("event data"), error in=w569) -> ()  [unwired: 1 in, 2 out]
          }
        }
      }
      frame Error {
        # "Return true in any case that should stop the loop."
      }
    }
  }
  n316 = Release Queue(queue=w44, error in (no error)=w46) -> (error out=w34:errorcluster)  [unwired: 1 in, 2 out]
  n317 = Unregister For Events(event registration refnum=w33, error in=w34) -> (error out=w19:errorcluster)
  n318 = Release Queue(queue=w18, error in (no error)=w19) -> ()  [unwired: 1 in, 3 out]
